vi "RichToFlatnise_DisconnectInfo.vi"(5 "OutputClusterType":T1, 11 "InputCluster":T3) -> (3 "OutputCluster":T1)   [LabVIEW 2021, in "basic_switch_executive_driver_client.lvlib"]
uses:
  basic_switch_executive_driver_client.lvlib
  nise_DisconnectInfo.ctl
  nise_SessionInformation.ctl
  <vilib>/Plug-In SDKs/Clients/Session Management V1/Session Reservation/Initialize and Close Session Behavior.ctl
  nise_DisconnectInfo_Flat.ctl
  nise_SessionInformation_Flat.ctl
  <vilib>/Plug-In SDKs/Clients/Session Management V1/Session Reservation/Session Reservation.lvclass
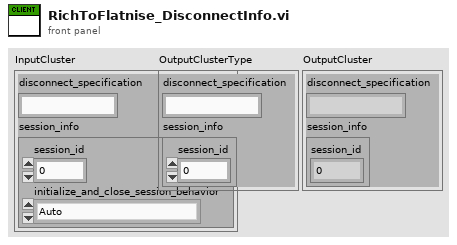
[diagram p1: front panel]
types:
  T1 = typedef "basic_switch_executive_driver_client.lvlib/nise_DisconnectInfo_Flat.ctl" = cluster{"disconnect_specification":string, "session_info":T2}
  T2 = typedef "basic_switch_executive_driver_client.lvlib/nise_SessionInformation_Flat.ctl" = cluster{"session_id":u32}
  T3 = typedef "basic_switch_executive_driver_client.lvlib/nise_DisconnectInfo.ctl" = cluster{"disconnect_specification":string, "session_info":T4}
  T4 = typedef "basic_switch_executive_driver_client.lvlib/nise_SessionInformation.ctl" = cluster{"session_id":u32, "initialize_and_close_session_behavior":T5}
  T5 = typedef "NI Session Management V1 Client.lvlib/Session Reservation.lvclass/Initialize and Close Session Behavior.ctl" = enum16{"Auto", "Initialize and Close", "Attach and Detach", "Initialize and Detach", "Attach and Close"}
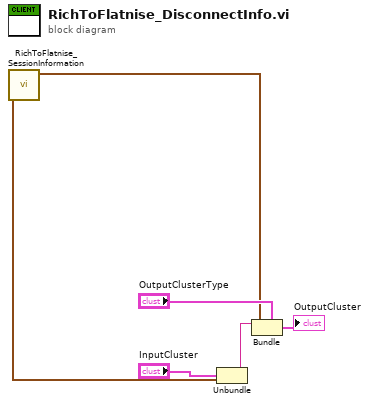
[diagram p0: block diagram]
diagram:
  n1 = Unbundle "Unbundle"("InputCluster") -> ("disconnect_specification"=w3:string, "session_info"=w2:T4)
  n2 = call "RichToFlatnise_SessionInformation.vi"("InputCluster"=w2) -> ("OutputCluster"=w1:T2)  [unwired: 10 in]
  n3 = Bundle "Bundle"(cluster="OutputClusterType", "disconnect_specification"=w3, "session_info"=w1) -> (→"OutputCluster":T1)
